vi "niFPGA I64xU16 - MSB.vi"(2 "A":i64, 3 "B":u16) -> (7 "A*B [Hi I64]":i64=2838 format="%08x")   [LabVIEW 2017]
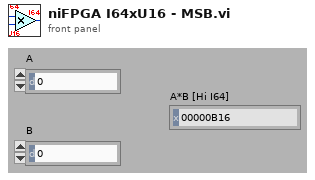
[diagram p1: front panel]
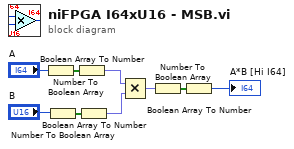
[diagram p0: block diagram]
diagram:
  n1 = Number To Boolean Array(number="A") -> (Boolean array=w7:bool[])
  n2 = Number To Boolean Array(number="B") -> (Boolean array=w8:bool[])
  n3 = Boolean Array To Number(Boolean array=w7) -> (number=w5:fxp<+/-,64,0>)
  n4 = Boolean Array To Number(Boolean array=w8) -> (number=w4:fxp<+,16,0>)
  n5 = Multiply(x=w5, y=w4) -> (x*y=w2:fxp<+/-,64,0>)
  n6 = Number To Boolean Array(number=w2) -> (Boolean array=w3:bool[])
  n7 = Boolean Array To Number(Boolean array=w3) -> (number=→"A*B [Hi I64]":i64)
